vi "TDS DCPS Readback.vi"(8 "error in (no error)":errorcluster, 10 "Signal InstConfig":string, 11 "Address":string) -> (0 "error out":errorcluster, 3 "Readback Values":T1)   [LabVIEW 2025, in "Interface Functions.lvlib"]
uses:
  Interface Functions.lvlib
panel:
  # "DCPS Readback"
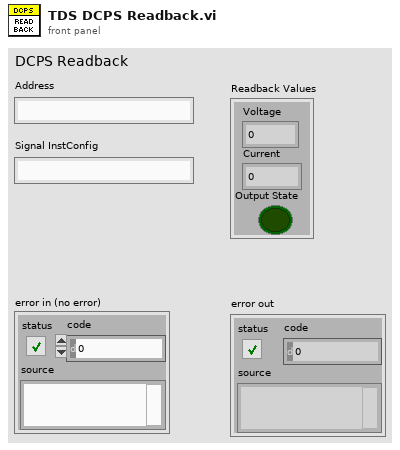
[diagram p1: front panel]
types:
  T1 = cluster{"Voltage":dbl, "Current":dbl, "Output State":bool}
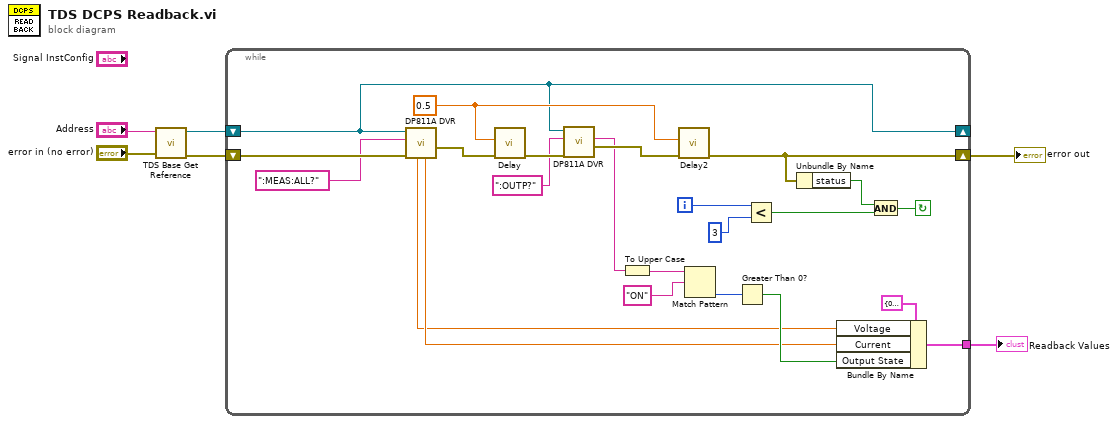
[diagram p0: block diagram]
diagram:
  n1 = call "TDS Base Get Reference.vi"("error in (no error)"="error in (no error)", "Address"="Address") -> ("error out"=w4:errorcluster, "Reference"=w3:refnum<visa-resource-name>)  [unwired: 8 in]
  n2 = while {
    shift-right: [w20] -> w2
    shift-left: w4 -> [w24]
    shift-right: [w16] -> _
    shift-left: w3 -> [w16]
    tunnel: [w7] -> w1
    i -> [w29]
    stop <- w25 continue-if-true
    w19 = 0.5 ("Delay Time (s)")
    n3 = call "DP811A DVR.vi"("error in (no error)"=w24, "write buffer"=":MEAS:ALL?", "VISA resource name"=w16) -> ("error out"=w23:errorcluster, "Current"=w9:dbl, "Voltage"=w8:dbl)  [unwired: 3 in, 3 out]
    n4 = call "Delay"("error in (no error)"=w23, "Delay Time (s)"=w19) -> ("error out"=w22:errorcluster)  [unwired: 9 in]
    n5 = call "DP811A DVR.vi"("error in (no error)"=w22, "write buffer"=":OUTP?", "VISA resource name"=w16) -> ("error out"=w21:errorcluster, "read buffer"=w12:string)  [unwired: 3 in, 4 out]
    n6 = To Upper Case(1:w12) -> (0:w15:string)
    n7 = call "Delay2"("error in (no error)"=w21, "Delay Time (s)"=w19) -> ("error out"=w20:errorcluster)  [unwired: 9 in]
    n8 = Match Pattern(string=w15, regular expression="ON") -> (offset past match=w14:i32)  [unwired: 1 in, 3 out]
    n9 = Greater Than 0?(x=w14) -> (x > 0?=w10:bool)
    n10 = Less?(x=w29, y=3) -> (x < y?=w26:bool)
    n11 = Unbundle By Name(w20) -> ("status"=w27:bool)
    n12 = Bundle By Name(cluster=T1 {"Voltage"=0.0, "Current"=0.0, "Output State"=FALSE} ("Readback Values"), "Voltage"=w8, "Current"=w9, "Output State"=w10) -> (w7:T1)
    n13 = And(x=w27, y=w26) -> (x .and. y?=w25:bool)
  }
  "error out" <- w2
  "Readback Values" <- w1
